vi "流程日志字段定义.vi"(7 "table输入":string, 11 "data in":T1) -> (1 "table输出":string, 2 "columns":string[](array[string]), 3 "data out":T1)   [LabVIEW 2016, in "PLC.lvlib"]
uses:
  PLC.lvlib
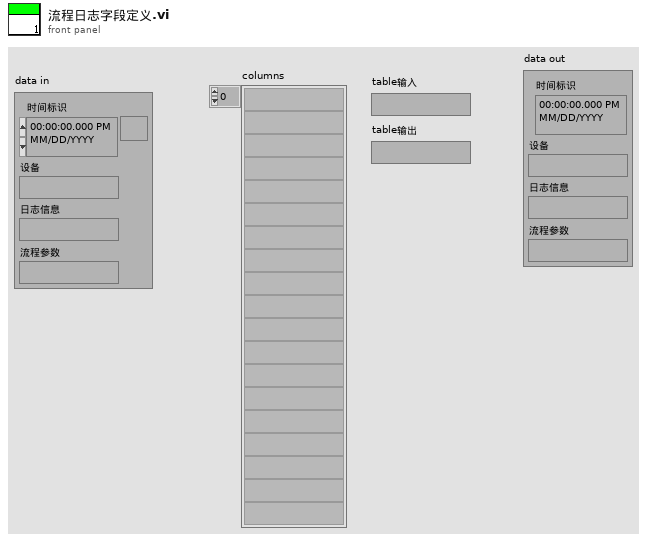
[diagram p1: front panel]
types:
  T1 = cluster{"时间标识":timestamp, "设备":string, "日志信息":string, "流程参数":string}
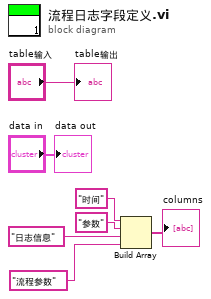
[diagram p0: block diagram]
diagram:
  n1 = Build Array("时间", "参数" ("元素"), "日志信息", "流程参数") -> (→"columns":string[])
  "table输出" <- "table输入"
  "data out" <- "data in"
